vi "在表格最后插入行.vi"(8 "错误输入（无错误）":errorcluster, 10 "内容":string[](array[string]), 11 "引用输入":refnum<vi>) -> (0 "错误输出":errorcluster, 3 "引用输出":refnum<vi>)   [LabVIEW 2014, in "表格.lvlib"]
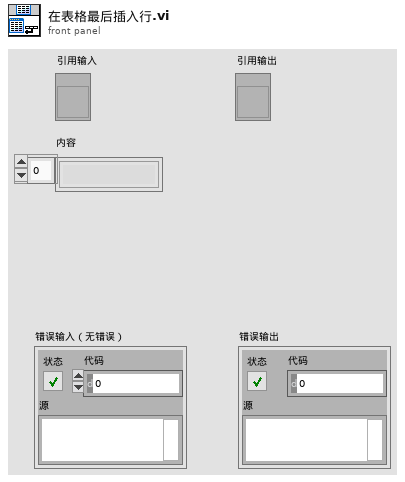
[diagram p1: front panel]
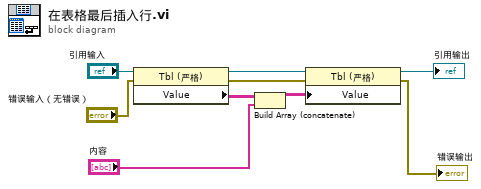
[diagram p0: block diagram]
diagram:
  n1 = property class="Tbl (严格)"(reference="引用输入", error in="错误输入（无错误）") -> (reference out=w6:refnum<vi>, error out=w5:errorcluster, "Value"=w8:string[][])
  n2 = Build Array (concatenate)(w8, "内容") -> (w4:string[][])
  n3 = property class="Tbl (严格)"(reference=w6, error in=w5, "Value"=w4) -> (reference out=→"引用输出":refnum<vi>, error out=→"错误输出":errorcluster)
